vi "Autonomous Independent.vi"() -> ()   [LabVIEW 2015]
doc: "This VI is called when autonomous begins, and will automatically be terminated when autonomous ends. You can carry out timed or sensor driven robot movement independently without needing to return to the caller."
uses:
  <vilib>/Rock Robotics/WPI/Solenoid/WPI_SolenoidValue.ctl
  <vilib>/Rock Robotics/WPI/Utilities/WPI_GetSetVariantRefNum.vi
  <vilib>/Rock Robotics/Network Tables/NT Read String.vi
  <vilib>/Rock Robotics/WPI/Solenoid/WPI_SolenoidSetEnum.vi
  <vilib>/Rock Robotics/Network Tables/NT Write Numeric Array.vi
  <vilib>/Rock Robotics/Network Tables/NT Write Boolean.vi
panel:
  out "Current Movement, for debugging":T1 {"Y Joystick Value" scale=1.0..-1.0; "X Joystick Value" scale=-1.0..1.0}
  in  "Array of robot movements":T2(array[cluster])=[{"X Joystick Value"=0.39393939393939403, "Y Joystick Value"=0.0, "Delay (sec)"=1.0, "Movement Name"="turn"}, {"X Joystick Value"=-0.3737373737373737, "Y Joystick Value"=0.0, "Delay (sec)"=1.0, "Movement Name"="turn back"}] {"Y Joystick Value" scale=1.0..-1.0; "X Joystick Value" scale=-1.0..1.0}
  # "Be sure to right-click and choose Data Operations>>Make Current Value default if you want to save the array values with the VI"
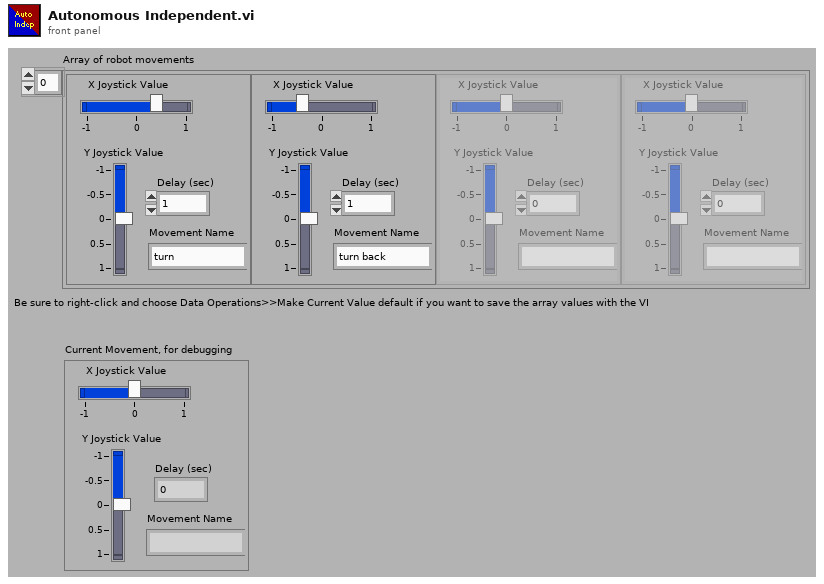
[diagram p1: front panel]
types:
  T1 = cluster{"X Joystick Value":dbl, "Y Joystick Value":dbl, "Delay (sec)":dbl, "Movement Name":string}
  T2 = cluster{"X Joystick Value":dbl, "Y Joystick Value":dbl, "Delay (sec)":dbl, "Movement Name":string}[]
  T3 = typedef "WPI_JoystickDevRef.ctl" = cluster{"Device":T4}
  T4 = typedef "WPI_JoystickDeviceEnum.ctl" = enum16{"USB 0", "USB 1", "USB 2", "USB 3", "USB 4", "USB 5"}
  T5 = typedef "WPI_SolenoidValue.ctl" = enum16{"Off", "On", "Forward", "Reverse"}
  T6 = typedef "WPI_SolenoidDevRef.ctl" = cluster{"DevStatus":errorcluster, "Pneumatics Control Module":u8, "Forward Solenoid Channel":T7, "Reverse Solenoid Channel":T7}
  T7 = typedef "WPI_SolenoidChannel.ctl" = enum8{"Solenoid 0", "Solenoid 1", "Solenoid 2", "Solenoid 3", "Solenoid 4", "Solenoid 5", "Solenoid 6", "Solenoid 7", "Invalid"}
  T8 = typedef "WPI_MotorControlDeviceRef.ctl" = cluster{"DeviceStatus":errorcluster, "Type":T9, "PWM":cluster{"PWM Channel":T10, "DeadBand":T11}, "CAN":cluster{"Device Number":u8, "Control Mode":T12, "Semaphore":T13, "Max Vout":dbl, "TalonSRX Control Mode":T14}, "Invert":bool}
  T9 = typedef "WPI_MotorControlType.ctl" = enum16{"PWM", "CAN", "CANTalonSRX"}
  T10 = typedef "FPGA_DIOPWMChannel.ctl" = enum8{"PWM 0", "PWM 1", "PWM 2", "PWM 3", "PWM 4", "PWM 5", "PWM 6", "PWM 7", "PWM 8", "PWM 9", "PWM MXP 0", "PWM MXP 1", "PWM MXP 2", "PWM MXP 3", "PWM MXP 4", "PWM MXP 5", "PWM MXP 6", "PWM MXP 7", "PWM MXP 8", "PWM MXP 9", "Invalid"}
  T11 = typedef "WPI_PWMDeadband.ctl" = cluster{"Name":string, "maxPositivePwm":i32, "minPositivePwm":i32, "centerPwm":i32, "maxNegativePwm":i32, "minNegativePwm":i32, "angularRange":u16}
  T12 = typedef "WPI_CANJaguar_ControlMode.ctl" = enum8{"Percent VBus", "Current", "Speed", "Position", "Voltage"}
  T13 = typedef "Semaphore RefNum" = refnum<k1>
  T14 = typedef "WPI_CANTalonSRX_APIControlMode.ctl" = enum8{"Percent VBus", "Speed", "Position", "Slave", "Unchanged / Invalid", "Voltage Compensation", "Current", "Motion Profile"}
  T15 = typedef "WPI_RobotDriveDevRef.ctl" = cluster{"DevStatus":errorcluster, "Motors[]":T8[], "Square Inputs":bool, "Max Output":dbl}
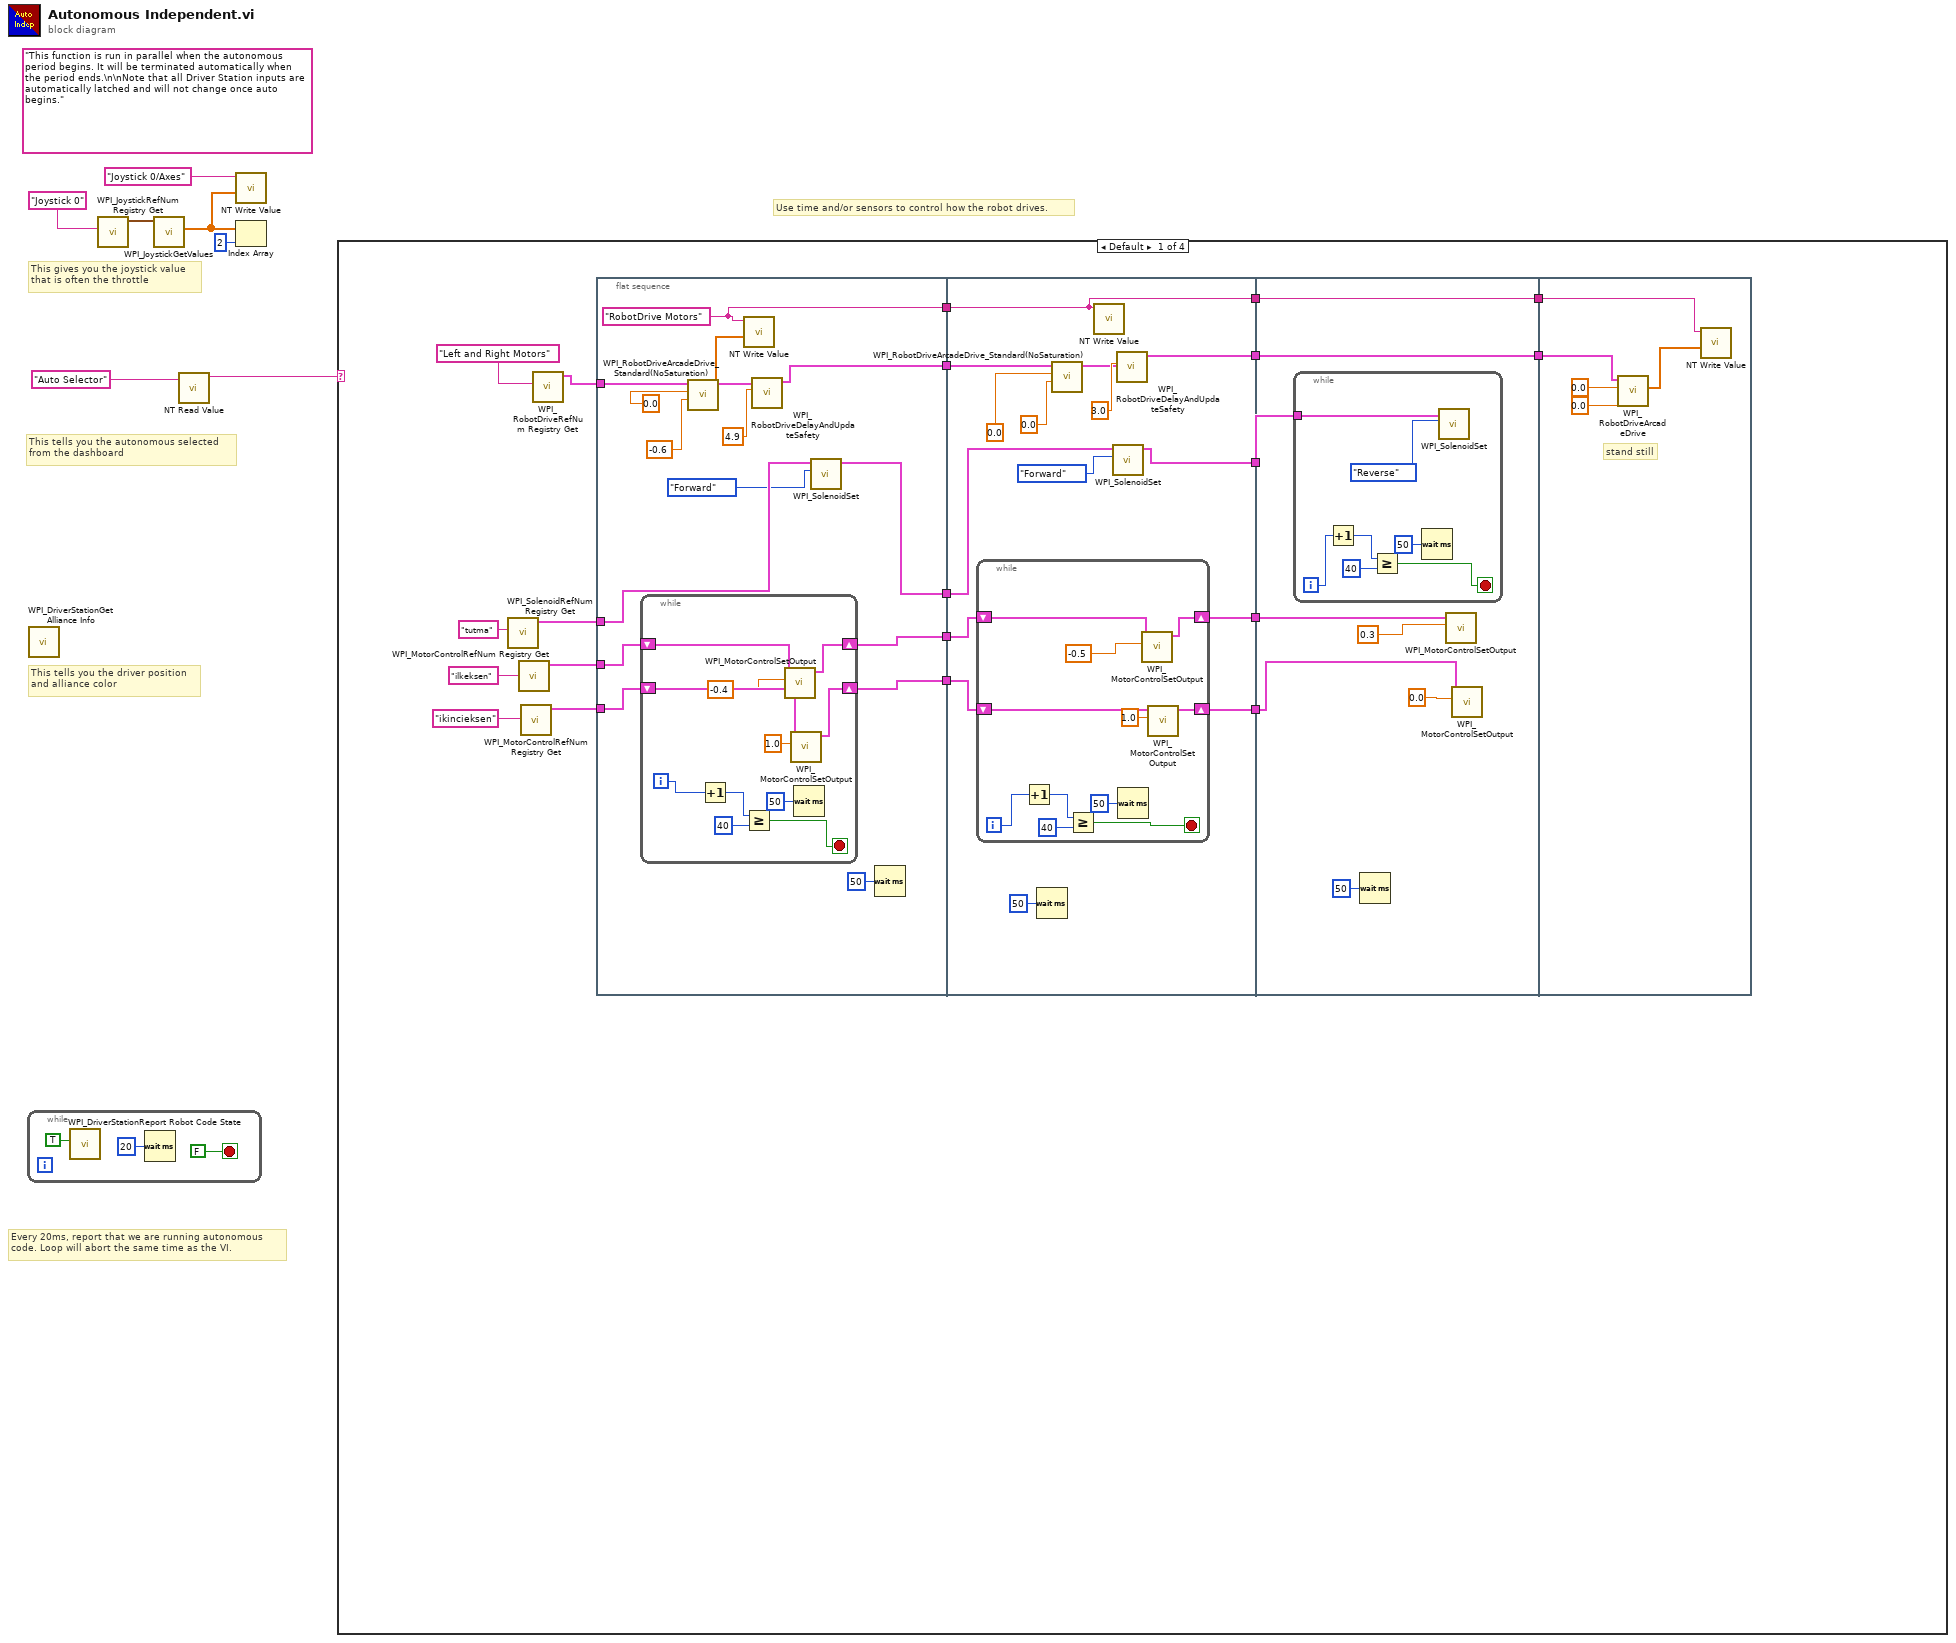
[diagram p0: block diagram]
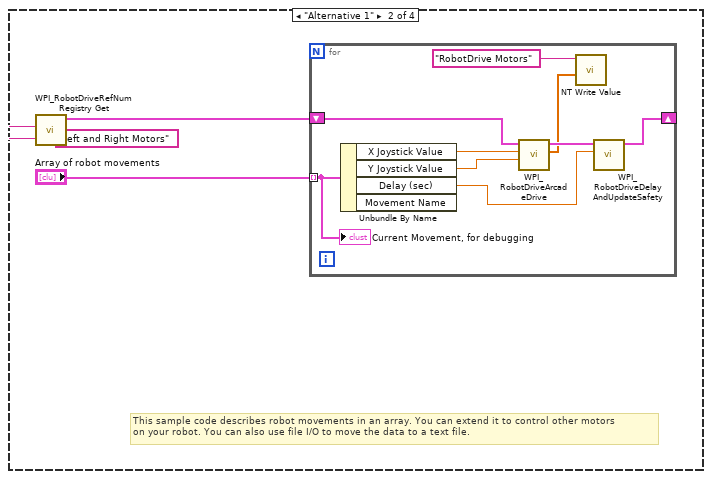
[diagram p2: hidden frame]
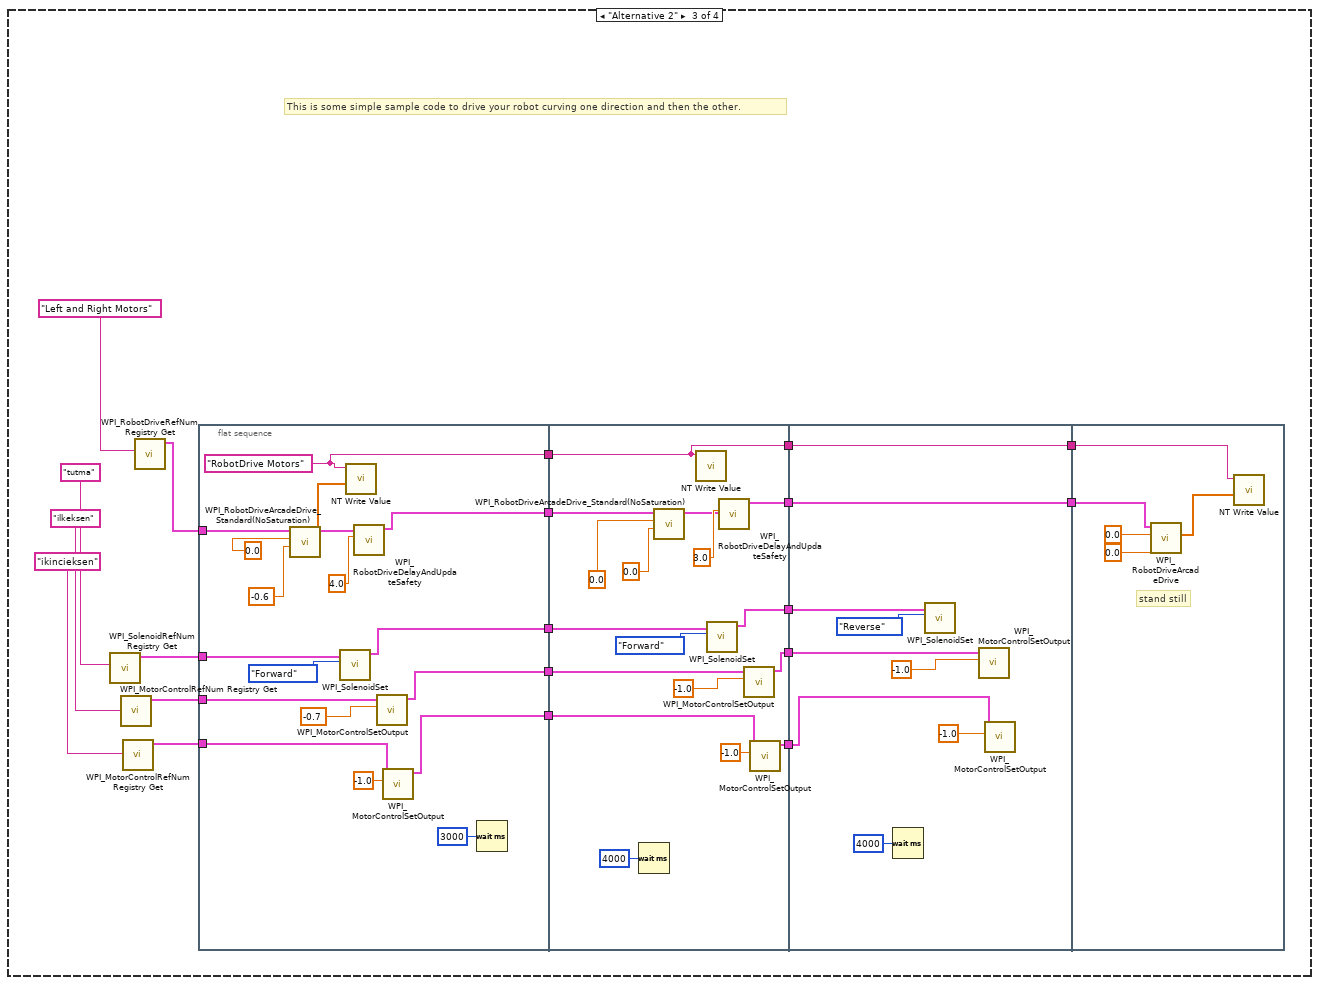
[diagram p3: hidden frame]
diagram:
  (unwired) "This function is run in parallel when the autonomous period begins. It will be terminated automatically when the period ends.\n\nNote that all Driver Station inputs are automatically latched and will not change once auto begins."
  # "This tells you the autonomous selected\nfrom the dashboard"
  # "Every 20ms, report that we are running autonomous\ncode. Loop will abort the same time as the VI."
  # "This gives you the joystick value\nthat is often the throttle"
  # "Use time and/or sensors to control how the robot drives."
  # "This tells you the driver position\nand alliance color"
  n1 = while {
    stop <- FALSE stop-if-true
    n2 = call <vilib>:"WPI_DriverStationReport Robot Code State.vi"("Autonomous"=TRUE) -> ()  [unwired: 10 in, 1 out]
    n3 = Wait (ms)(milliseconds to wait=u32 20) -> ()  [unwired: 1 out]
  }
  n4 = call <vilib>:"WPI_DriverStationGet Alliance Info.vi"() -> ()  [unwired: 12 out]
  n5 = call <vilib>:"WPI_JoystickRefNum Registry Get.vi"("refnum name"="Joystick 0") -> ("JoystickDevRef"=w6:T3)  [unwired: 1 in, 9 out]
  n6 = call <vilib>:"WPI_JoystickGetValues.vi"("JoystickDevRef"=w6) -> ("Axes"=w2:dbl[])  [unwired: 6 in, 4 out]
  n7 = call-poly <vilib>:"NT Read Value.vi"("Name"="Auto Selector") -> ("String"=w3:string)  [unwired: 9 in, 1 out]
  n8 = call-poly <vilib>:"NT Write Value.vi"("Numeric Array"=w2, "Name"="Joystick 0/Axes") -> ()  [unwired: 9 in, 1 out]
  n9 = Index Array(array=w2, index=2) -> ()  [unwired: 1 out]
  n10 = case shown="Default" w3 {
    frame Default {
      n11 = call <vilib>:"WPI_SolenoidRefNum Registry Get.vi"("refnum name"="tutma") -> ("SolenoidDevRef"=w13:T6)  [unwired: 9 in, 1 out]
      n12 = call <vilib>:"WPI_MotorControlRefNum Registry Get.vi"("refnum name"="ilkeksen") -> ("MotorControlDevRef"=w12:T8)  [unwired: 9 in, 1 out]
      n13 = call <vilib>:"WPI_MotorControlRefNum Registry Get.vi"("refnum name"="ikincieksen") -> ("MotorControlDevRef"=w11:T8)  [unwired: 9 in, 1 out]
      n14 = call <vilib>:"WPI_RobotDriveRefNum Registry Get.vi"("refnum name"="Left and Right Motors") -> ("RobotDriveDevRef"=w14:T15)  [unwired: 1 in, 9 out]
      n15 = flat-sequence {
        tunnel: w14 -> [w41]
        tunnel: [w40] -> w30
        tunnel: [w39] -> w29
        tunnel: w13 -> [w32]
        tunnel: w12 -> [w38]
        tunnel: w11 -> [w37]
        tunnel: [w33] -> w28
        tunnel: [w35] -> w27
        tunnel: [w34] -> w26
        tunnel: w30 -> [w68]
        tunnel: w29 -> [w67]
        tunnel: [w67] -> w25
        tunnel: [w65] -> w24
        tunnel: w28 -> [w60]
        tunnel: w27 -> [w64]
        tunnel: w26 -> [w63]
        tunnel: [w58] -> w23
        tunnel: [w62] -> w22
        tunnel: [w61] -> w21
        tunnel: w25 -> [w91]
        tunnel: [w91] -> w20
        tunnel: w24 -> [w90]
        tunnel: [w90] -> w19
        tunnel: w23 -> [w87]
        tunnel: w22 -> [w86]
        tunnel: w21 -> [w85]
        tunnel: w20 -> [w100]
        tunnel: w19 -> [w99]
        frame #0 {
          w39 = "RobotDrive Motors" ("Name")
          n16 = while {
            shift-right: [w53] -> w35
            shift-left: w38 -> [w57]
            shift-right: [w52] -> w34
            shift-left: w37 -> [w56]
            i -> [w51]
            stop <- w49 stop-if-true
            n17 = Increment(x=w51) -> (x+1=w50:i32)
            n18 = Greater Or Equal?(x=w50, y=40) -> (x >= y?=w49:bool)
            n19 = call <vilib>:"WPI_MotorControlSetOutput.vi"("Output"=-0.4, "MotorControlDevRef"=w57) -> ("MotorControlDevRef"=w53:T8)  [unwired: 7 in, 2 out]
            n20 = call <vilib>:"WPI_MotorControlSetOutput.vi"("Output"=1.0, "MotorControlDevRef"=w56) -> ("MotorControlDevRef"=w52:T8)  [unwired: 7 in, 2 out]
            n21 = Wait (ms)(milliseconds to wait=u32 50) -> ()  [unwired: 1 out]
          }
          n22 = call <vilib>:"WPI_RobotDriveArcadeDrive_Standard(NoSaturation).vi"("Y axis value"=-0.6, "X axis value"=0.0, "RobotDriveDevRef"=w41) -> ("Motor Values"=w42:dbl[], "RobotDriveDevRef"=w45:T15)  [unwired: 1 in, 6 out]
          n23 = call-poly <vilib>:"NT Write Value.vi"("Numeric Array"=w42, "Name"=w39) -> ()  [unwired: 9 in, 1 out]
          n24 = call <vilib>:"WPI_RobotDriveDelayAndUpdateSafety.vi"("Delay (s)"=4.9, "RobotDriveDevRef"=w45) -> ("RobotDriveDevRef 2"=w40:T15)  [unwired: 8 in, 1 out]
          n25 = call-poly <vilib>:"WPI_SolenoidSet.vi"("Value"=WPI_SolenoidValue."Forward", "SolenoidDevRef"=w32) -> ("SolenoidDevRef"=w33:T6)  [unwired: 8 in, 1 out]
          n26 = Wait (ms)(milliseconds to wait=u32 50) -> ()  [unwired: 1 out]
        }
        frame #1 {
          n27 = while {
            shift-right: [w79] -> w62
            shift-left: w64 -> [w81]
            shift-right: [w78] -> w61
            shift-left: w63 -> [w80]
            i -> [w73]
            stop <- w74 stop-if-true
            n28 = Increment(x=w73) -> (x+1=w77:i32)
            n29 = Greater Or Equal?(x=w77, y=40) -> (x >= y?=w74:bool)
            n30 = Wait (ms)(milliseconds to wait=u32 50) -> ()  [unwired: 1 out]
            n31 = call <vilib>:"WPI_MotorControlSetOutput.vi"("Output"=-0.5, "MotorControlDevRef"=w81) -> ("MotorControlDevRef"=w79:T8)  [unwired: 7 in, 2 out]
            n32 = call <vilib>:"WPI_MotorControlSetOutput.vi"("Output"=1.0, "MotorControlDevRef"=w80) -> ("MotorControlDevRef"=w78:T8)  [unwired: 7 in, 2 out]
          }
          n33 = Wait (ms)(milliseconds to wait=u32 50) -> ()  [unwired: 1 out]
          n34 = call <vilib>:"WPI_RobotDriveArcadeDrive_Standard(NoSaturation).vi"("Y axis value"=0.0, "X axis value"=0.0, "RobotDriveDevRef"=w68) -> ("RobotDriveDevRef"=w71:T15)  [unwired: 1 in, 7 out]
          n35 = call-poly <vilib>:"NT Write Value.vi"("Name"=w67) -> ()  [unwired: 10 in, 1 out]
          n36 = call-poly <vilib>:"WPI_SolenoidSet.vi"("Value"=WPI_SolenoidValue."Forward", "SolenoidDevRef"=w60) -> ("SolenoidDevRef"=w58:T6)  [unwired: 8 in, 1 out]
          n37 = call <vilib>:"WPI_RobotDriveDelayAndUpdateSafety.vi"("Delay (s)"=3.0, "RobotDriveDevRef"=w71) -> ("RobotDriveDevRef 2"=w65:T15)  [unwired: 8 in, 1 out]
        }
        frame #2 {
          n38 = while {
            tunnel: w87 -> [w97]
            i -> [w92]
            stop <- w93 stop-if-true
            n39 = Increment(x=w92) -> (x+1=w96:i32)
            n40 = Greater Or Equal?(x=w96, y=40) -> (x >= y?=w93:bool)
            n41 = Wait (ms)(milliseconds to wait=u32 50) -> ()  [unwired: 1 out]
            n42 = call-poly <vilib>:"WPI_SolenoidSet.vi"("Value"=WPI_SolenoidValue."Reverse", "SolenoidDevRef"=w97) -> ()  [unwired: 8 in, 2 out]
          }
          n43 = Wait (ms)(milliseconds to wait=u32 50) -> ()  [unwired: 1 out]
          n44 = call <vilib>:"WPI_MotorControlSetOutput.vi"("Output"=0.3, "MotorControlDevRef"=w86) -> ()  [unwired: 7 in, 3 out]
          n45 = call <vilib>:"WPI_MotorControlSetOutput.vi"("Output"=0.0, "MotorControlDevRef"=w85) -> ()  [unwired: 7 in, 3 out]
        }
        frame #3 {
          # "stand still"
          n46 = call-poly <vilib>:"WPI_RobotDriveArcadeDrive.vi"("Y axis value"=0.0, "X axis value"=0.0, "RobotDriveDevRef"=w99) -> ("Motor Values"=w101:dbl[])  [unwired: 1 in, 7 out]
          n47 = call-poly <vilib>:"NT Write Value.vi"("Numeric Array"=w101, "Name"=w100) -> ()  [unwired: 9 in, 1 out]
        }
      }
    }
    frame "Alternative 1" {
      # "This sample code describes robot movements in an array. You can extend it to control other motors\non your robot. You can also use file I/O to move the data to a text file."
      n48 = call <vilib>:"WPI_RobotDriveRefNum Registry Get.vi"("refnum name"="Left and Right Motors") -> ("RobotDriveDevRef"=w105:T15)  [unwired: 1 in, 9 out]
      n49 = for {
        shift-right: [w113] -> _
        shift-left: w105 -> [w114]
        tunnel: "Array of robot movements" -> [w109] mode=indexing
        n50 = Unbundle By Name(w109) -> ("X Joystick Value"=w112:dbl, "Y Joystick Value"=w111:dbl, "Delay (sec)"=w110:dbl)  [unwired: 1 out]
        n51 = call-poly <vilib>:"WPI_RobotDriveArcadeDrive.vi"("Y axis value"=w111, "X axis value"=w112, "RobotDriveDevRef"=w114) -> ("Motor Values"=w107:dbl[], "RobotDriveDevRef"=w115:T15)  [unwired: 1 in, 6 out]
        n52 = call-poly <vilib>:"NT Write Value.vi"("Numeric Array"=w107, "Name"="RobotDrive Motors") -> ()  [unwired: 9 in, 1 out]
        n53 = call <vilib>:"WPI_RobotDriveDelayAndUpdateSafety.vi"("Delay (s)"=w110, "RobotDriveDevRef"=w115) -> ("RobotDriveDevRef 2"=w113:T15)  [unwired: 8 in, 1 out]
        "Current Movement, for debugging" <- w109
      }
    }
    frame "Alternative 2" {
      # "This is some simple sample code to drive your robot curving one direction and then the other."
      n54 = call <vilib>:"WPI_SolenoidRefNum Registry Get.vi"("refnum name"="tutma") -> ("SolenoidDevRef"=w128:T6)  [unwired: 9 in, 1 out]
      n55 = call <vilib>:"WPI_MotorControlRefNum Registry Get.vi"("refnum name"="ilkeksen") -> ("MotorControlDevRef"=w127:T8)  [unwired: 9 in, 1 out]
      n56 = call <vilib>:"WPI_MotorControlRefNum Registry Get.vi"("refnum name"="ikincieksen") -> ("MotorControlDevRef"=w126:T8)  [unwired: 9 in, 1 out]
      n57 = call <vilib>:"WPI_RobotDriveRefNum Registry Get.vi"("refnum name"="Left and Right Motors") -> ("RobotDriveDevRef"=w131:T15)  [unwired: 1 in, 9 out]
      n58 = flat-sequence {
        tunnel: w131 -> [w148]
        tunnel: [w147] -> w130
        tunnel: [w146] -> w129
        tunnel: w128 -> [w145]
        tunnel: w127 -> [w144]
        tunnel: w126 -> [w143]
        tunnel: [w138] -> w121
        tunnel: [w137] -> w120
        tunnel: [w136] -> w119
        tunnel: w130 -> [w166]
        tunnel: w129 -> [w165]
        tunnel: [w165] -> w125
        tunnel: [w163] -> w123
        tunnel: w121 -> [w159]
        tunnel: w120 -> [w158]
        tunnel: w119 -> [w157]
        tunnel: [w156] -> w118
        tunnel: [w155] -> w117
        tunnel: [w154] -> w116
        tunnel: w125 -> [w179]
        tunnel: [w179] -> w124
        tunnel: w123 -> [w178]
        tunnel: [w178] -> w122
        tunnel: w118 -> [w174]
        tunnel: w117 -> [w173]
        tunnel: w116 -> [w172]
        tunnel: w124 -> [w181]
        tunnel: w122 -> [w180]
        frame #0 {
          w146 = "RobotDrive Motors" ("Name")
          n59 = call <vilib>:"WPI_RobotDriveArcadeDrive_Standard(NoSaturation).vi"("Y axis value"=-0.6, "X axis value"=0.0, "RobotDriveDevRef"=w148) -> ("Motor Values"=w149:dbl[], "RobotDriveDevRef"=w152:T15)  [unwired: 1 in, 6 out]
          n60 = call-poly <vilib>:"WPI_SolenoidSet.vi"("Value"=WPI_SolenoidValue."Forward", "SolenoidDevRef"=w145) -> ("SolenoidDevRef"=w138:T6)  [unwired: 8 in, 1 out]
          n61 = call-poly <vilib>:"NT Write Value.vi"("Numeric Array"=w149, "Name"=w146) -> ()  [unwired: 9 in, 1 out]
          n62 = call <vilib>:"WPI_RobotDriveDelayAndUpdateSafety.vi"("Delay (s)"=4.0, "RobotDriveDevRef"=w152) -> ("RobotDriveDevRef 2"=w147:T15)  [unwired: 8 in, 1 out]
          n63 = call <vilib>:"WPI_MotorControlSetOutput.vi"("Output"=-0.7, "MotorControlDevRef"=w144) -> ("MotorControlDevRef"=w137:T8)  [unwired: 7 in, 2 out]
          n64 = call <vilib>:"WPI_MotorControlSetOutput.vi"("Output"=-1.0, "MotorControlDevRef"=w143) -> ("MotorControlDevRef"=w136:T8)  [unwired: 7 in, 2 out]
          n65 = Wait (ms)(milliseconds to wait=u32 3000) -> ()  [unwired: 1 out]
        }
        frame #1 {
          n66 = Wait (ms)(milliseconds to wait=u32 4000) -> ()  [unwired: 1 out]
          n67 = call <vilib>:"WPI_RobotDriveArcadeDrive_Standard(NoSaturation).vi"("Y axis value"=0.0, "X axis value"=0.0, "RobotDriveDevRef"=w166) -> ("RobotDriveDevRef"=w169:T15)  [unwired: 1 in, 7 out]
          n68 = call-poly <vilib>:"NT Write Value.vi"("Name"=w165) -> ()  [unwired: 10 in, 1 out]
          n69 = call-poly <vilib>:"WPI_SolenoidSet.vi"("Value"=WPI_SolenoidValue."Forward", "SolenoidDevRef"=w159) -> ("SolenoidDevRef"=w156:T6)  [unwired: 8 in, 1 out]
          n70 = call <vilib>:"WPI_RobotDriveDelayAndUpdateSafety.vi"("Delay (s)"=3.0, "RobotDriveDevRef"=w169) -> ("RobotDriveDevRef 2"=w163:T15)  [unwired: 8 in, 1 out]
          n71 = call <vilib>:"WPI_MotorControlSetOutput.vi"("Output"=-1.0, "MotorControlDevRef"=w158) -> ("MotorControlDevRef"=w155:T8)  [unwired: 7 in, 2 out]
          n72 = call <vilib>:"WPI_MotorControlSetOutput.vi"("Output"=-1.0, "MotorControlDevRef"=w157) -> ("MotorControlDevRef"=w154:T8)  [unwired: 7 in, 2 out]
        }
        frame #2 {
          n73 = Wait (ms)(milliseconds to wait=u32 4000) -> ()  [unwired: 1 out]
          n74 = call-poly <vilib>:"WPI_SolenoidSet.vi"("Value"=WPI_SolenoidValue."Reverse", "SolenoidDevRef"=w174) -> ()  [unwired: 8 in, 2 out]
          n75 = call <vilib>:"WPI_MotorControlSetOutput.vi"("Output"=-1.0, "MotorControlDevRef"=w173) -> ()  [unwired: 7 in, 3 out]
          n76 = call <vilib>:"WPI_MotorControlSetOutput.vi"("Output"=-1.0, "MotorControlDevRef"=w172) -> ()  [unwired: 7 in, 3 out]
        }
        frame #3 {
          # "stand still"
          n77 = call-poly <vilib>:"WPI_RobotDriveArcadeDrive.vi"("Y axis value"=0.0, "X axis value"=0.0, "RobotDriveDevRef"=w180) -> ("Motor Values"=w182:dbl[])  [unwired: 1 in, 7 out]
          n78 = call-poly <vilib>:"NT Write Value.vi"("Numeric Array"=w182, "Name"=w181) -> ()  [unwired: 9 in, 1 out]
        }
      }
    }
    frame "Your Turn" {
    }
  }
